vi "PH_FIFORead.vi"(0 "Device Index":i32, 5 "Buffer In":u32[](array[numeric]), 7 "Count":u32, 11 "error in (no error)":errorcluster) -> (4 "OK":bool, 6 "Buffer Out":u32[](array[numeric]), 8 "Data Count":i32, 14 "FiFo Overrun":bool, 15 "error out":errorcluster)   [LabVIEW 2010]
uses:
  PHLib.dll
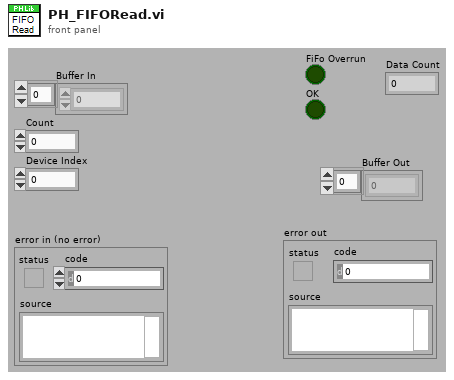
[diagram p1: front panel]
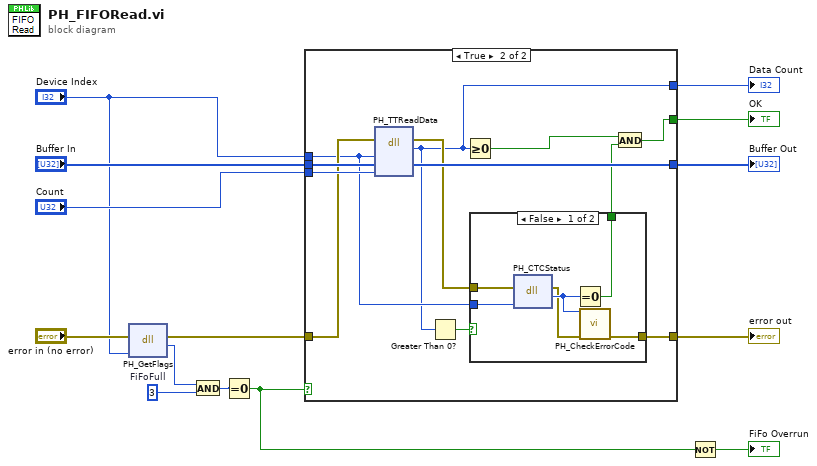
[diagram p0: block diagram]
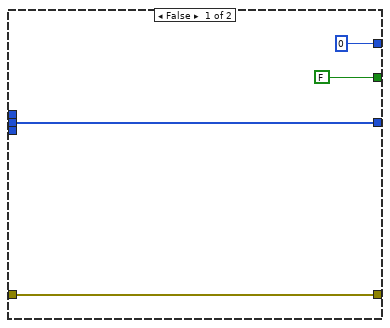
[diagram p2: hidden frame]
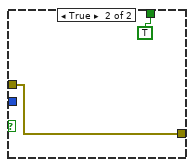
[diagram p3: hidden frame]
diagram:
  w10 = 3  # FiFoFull
  n1 = dll-call lib="C:/LabVIEW Programs/MT Scan PicoHarp/SubVIs/PHLib.dll" fn="PH_GetFlags"(error in="error in (no error)", "devidx"="Device Index") -> (error out=w4:errorcluster, "return type"=w8:i32)  [unwired: 3 in, 1 out]
  n2 = And(x=w8, y=w10) -> (x .and. y?=w9:i32)
  n3 = Equal To 0?(x=w9) -> (x = 0?=w7:bool)
  n4 = case shown="True" w7 {
    tunnel: "Buffer In" -> [w16 w30]
    tunnel: "Count" -> [_ w29]
    tunnel: "Device Index" -> [_ w23]
    tunnel: [FALSE ("OK") w25] -> w5
    tunnel: w4 -> [w17 w28]
    tunnel: [w17 w20] -> w3
    tunnel: [w16 w27] -> w2
    tunnel: [0 ("return type") w19] -> w1
    frame False {
    }
    frame True {
      n5 = dll-call lib="C:/LabVIEW Programs/MT Scan PicoHarp/SubVIs/PHLib.dll" fn="PH_TTReadData"(error in=w28, "devidx"=w23, "buffer"=w30, "count"=w29) -> (error out=w22:errorcluster, "return type"=w19:i32, "buffer"=w27:u32[])  [unwired: 4 in, 1 out]
      n6 = Greater Than 0?(x=w19) -> (x > 0?=w24:bool)
      n7 = Greater Or Equal To 0?(x=w19) -> (x >= 0?=w26:bool)
      n8 = case shown="False" w24 {
        tunnel: w23 -> [w36 _]
        tunnel: w22 -> [w35 w37]
        tunnel: [w34 TRUE] -> w21
        tunnel: [w31 w37] -> w20
        frame False {
          n9 = dll-call lib="C:/LabVIEW Programs/MT Scan PicoHarp/SubVIs/PHLib.dll" fn="PH_CTCStatus"(error in=w35, "devidx"=w36) -> (error out=w32:errorcluster, "return type"=w33:i32)  [unwired: 3 in, 1 out]
          n10 = Equal To 0?(x=w33) -> (x = 0?=w34:bool)
          n11 = call "PH_CheckErrorCode.vi"("errcode"=w33, "error in (no error)"=w32) -> ("error out"=w31:errorcluster)  [unwired: 12 in, 1 out]
        }
        frame True {
        }
      }
      n12 = And(x=w26, y=w21) -> (x .and. y?=w25:bool)
    }
  }
  "OK" <- w5
  "error out" <- w3
  "Buffer Out" <- w2
  "Data Count" <- w1
  n13 = Not ("CTCDone")(x=w7) -> (.not. x?=→"FiFo Overrun":bool)
